vi "ABR-Init Hardware.vi"(0 "Params":T1={"Stimulus"={"Destination"="", "Waveform"=enum."TONE PIP", "Frequency (kHz)"=16.0, "Rep rate (/sec)"=30.0, "Alternate Polarity"=FALSE, "Sampling rate (Hz)"=0.0, "Duration (ms)"=30.0, "Ramp (ms)"=5.0, "Click width (us)"=0.0, "ITI"=enum."Rate"}, "Sequence"={"Start (dB)"=20, "Stop (dB)"=80, "Step (dB)"=5}, "Response"={"CAP or ABR"=enum."ABR", "Gain"=10000, "Averages"=512, "Window (ms)"=8.5, "Thr Fast Steps"=8.5, "Fs (Hz)"=25000.0, "Save raw"=FALSE}, "Normalize"=FALSE, "Reject"=0.0} {"Sequence"."Start (dB)" step=5; "Response"."Thr Fast Steps" format="%.2f"; "Response"."Window (ms)" format="%.2f"; "Stimulus"."Frequency (kHz)" format="%.2f"}, 11 "error in (no error)":errorcluster) -> (4 "Runtime":T5, 6 "AO npts":i32, 8 "Coerced rep rate":dbl, 15 "error out":errorcluster)   [LabVIEW 2020]
uses:
  Typedefs/ABR-Runtime Data.ctl
  epl-vi-lib/Signal Synthesis VIs/4th Generation/Classes/SignalManager/SignalManager.lvclass
  Typedefs/ABR-Parameters.ctl
  Typedefs/ABR-Stimulus.ctl
  Typedefs/ABR-Sequence.ctl
  Typedefs/ABR-Response.ctl
  5664aaa6-f0d2-4dbe-9bd7-bb78e569ca1b.vi
  6bfe4fab-d2cc-4fad-8abc-22872ba60b63.vi
  0f633bf1-3711-4c41-a985-7e54c01dc944.vi
  5e16f318-188a-4eb5-81ba-3342a0d43969.vi
  <vilib>/Utility/config.llb/Open Config Data.vi
  <vilib>/Utility/config.llb/Get Key Names.vi
  <vilib>/Utility/config.llb/Read Key.vi
  <vilib>/Utility/config.llb/Read Key (String).vi
  epl-vi-lib/Utility VIs/Array Manipulation VIs/String Array to Comma Separated String.vi
  <vilib>/Utility/error.llb/Error Cluster From Error Code.vi
  <vilib>/Utility/config.llb/Close Config Data.vi
  epl-vi-lib/PXI DAQ VIs/AODO/AODO-Engine.vi
  epl-vi-lib/PXI DAQ VIs/AIDI/AIDI-Engine.vi
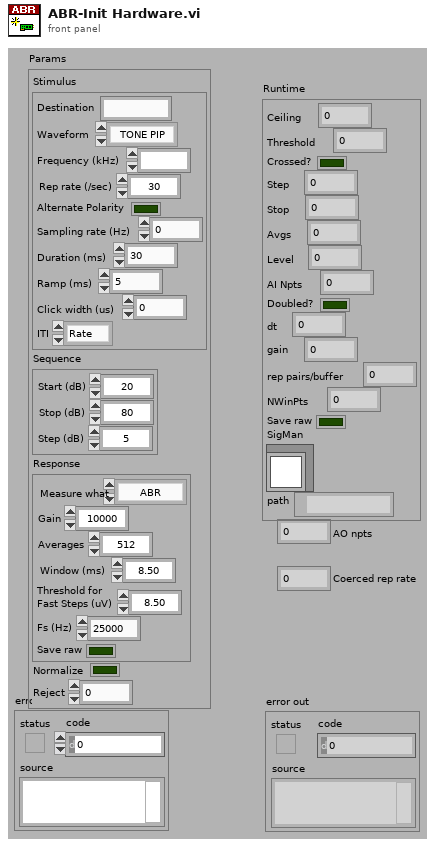
[diagram p1: front panel]
types:
  T1 = typedef "ABR-Parameters.ctl" = cluster{"Stimulus":T2, "Sequence":T3, "Response":T4, "Normalize":bool, "Reject":dbl}
  T2 = typedef "ABR-Stimulus.ctl" = cluster{"Destination":string, "Waveform":enum16{"TONE PIP", "CLICK"}, "Frequency (kHz)":ext, "Rep rate (/sec)":dbl, "Alternate Polarity":bool, "Sampling rate (Hz)":dbl, "Duration (ms)":dbl, "Ramp (ms)":dbl, "Click width (us)":dbl, "ITI":enum16{"Rate", "Interval"}}
  T3 = typedef "ABR-Sequence.ctl" = cluster{"Start (dB)":i32, "Stop (dB)":i32, "Step (dB)":i32}
  T4 = typedef "ABR-Response.ctl" = cluster{"CAP or ABR":enum16{"CAP", "ABR"}, "Gain":i32, "Averages":i32, "Window (ms)":sgl, "Thr Fast Steps":sgl, "Fs (Hz)":dbl, "Save raw":bool}
  T5 = typedef "ABR-Runtime Data.ctl" = cluster{"Ceiling":dbl, "Threshold":dbl, "Crossed?":bool, "Step":dbl, "Stop":i32, "Avgs":i32, "Level":dbl, "AI Npts":i32, "Doubled?":bool, "dt":dbl, "gain":dbl, "rep pairs/buffer":i32, "NWinPts":i32, "Save raw":bool, "SigMan":refnum<class "SignalManager.lvclass">, "path":path}
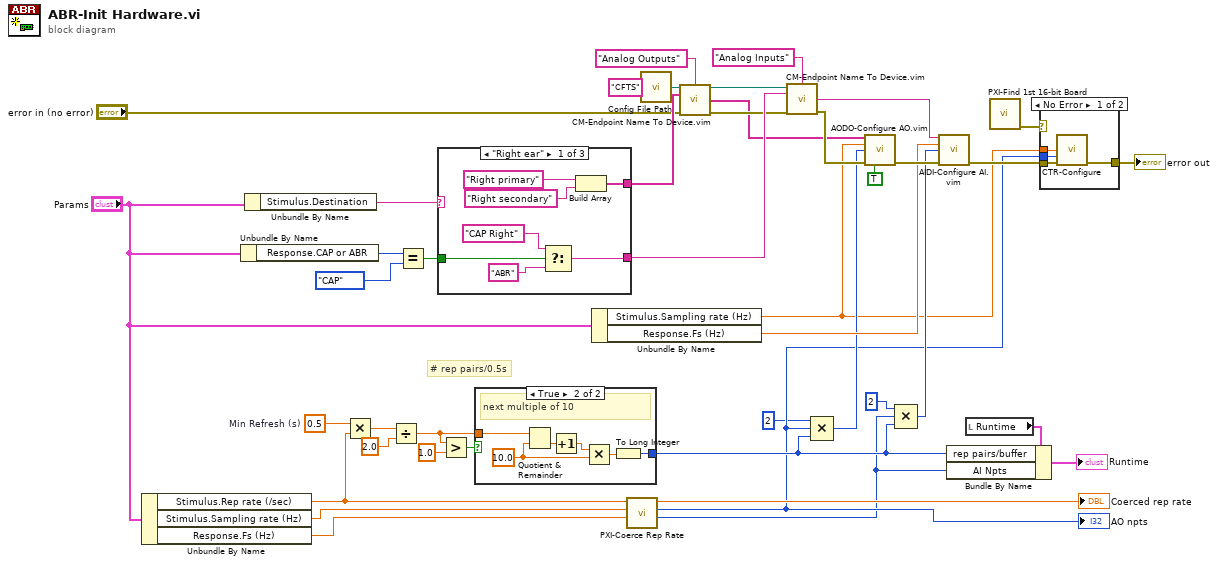
[diagram p0: block diagram]
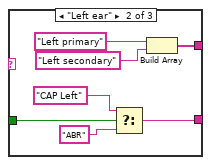
[diagram p3: hidden frame]
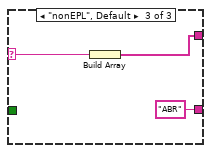
[diagram p4: hidden frame]
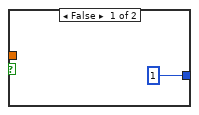
[diagram p5: hidden frame]
diagram:
  w35 = 0.5  # Min Refresh (s)
  # "# rep pairs/0.5s"
  n1 = Unbundle By Name("Params") -> ("Stimulus.Rep rate (/sec)"=w34:dbl, "Stimulus.Sampling rate (Hz)"=w14:dbl, "Response.Fs (Hz)"=w13:dbl)
  n2 = Unbundle By Name("Params") -> ("Response.CAP or ABR"=w31:enum16{"CAP", "ABR"})
  n3 = Unbundle By Name("Params") -> ("Stimulus.Destination"=w33:string)
  n4 = Multiply(x=w35, y=w34) -> (x*y=w36:dbl)
  n5 = Divide(x=w36, y=2.0) -> (x/y=w39:dbl)
  n6 = Equal?(x=w31, y=enum16{"CAP", "ABR"}."CAP") -> (x = y?=w29:bool)
  n7 = case shown="\"Right ear\"" w33 {
    selector: w33 -> [_ _ w60]
    tunnel: [w48 w55 w59] -> w23
    tunnel: w29 -> [w47 w54 _]
    tunnel: [w44 w51 "ABR"] -> w24
    frame "Right ear" {
      n8 = Select(t="CAP Right", s=w47, f="ABR") -> (s? t:f=w44:string)
      n9 = Build Array("Right primary", "Right secondary") -> (w48:string[])
    }
    frame "Left ear" {
      n10 = Select(t="CAP Left", s=w54, f="ABR") -> (s? t:f=w51:string)
      n11 = Build Array("Left primary", "Left secondary") -> (w55:string[])
    }
    frame "nonEPL", Default {
      n12 = Build Array(w60) -> (w59:string[])
    }
  }
  n13 = Greater?(x=w39, y=1.0) -> (0:w38:bool)
  n14 = case shown="True" w38 {
    tunnel: w39 -> [_ w67]
    tunnel: [1 w63] -> w11
    frame False {
    }
    frame True {
      w66 = 10.0 ("y")
      # "next multiple of 10"
      n15 = Quotient & Remainder(x=w67, y=w66) -> (floor(x/y)=w64:dbl)  [unwired: 1 out]
      n16 = Increment(x=w64) -> (x+1=w62:dbl)
      n17 = Multiply(x=w62, y=w66) -> (x*y=w65:dbl)
      n18 = To Long Integer(number=w65) -> (32bit integer=w63:i32)
    }
  }
  n19 = Unbundle By Name("Params") -> ("Stimulus.Sampling rate (Hz)"=w7:dbl, "Response.Fs (Hz)"=w15:dbl)
  n20 = call "PXI-Coerce Rep Rate.vi"("AI sampling rate (Hz)"=w13, "AO sampling rate (Hz)"=w14, "Rep rate (Hz)"=w34) -> ("AI npts"=w2:i32, "AO npts"=w6:i32, "Coerced rep rate (Hz)"=→"Coerced rep rate":dbl)  [unwired: 5 in, 1 out]
  "AO npts" <- w6
  n21 = call "Config File Path.vi"("AppName"="CFTS") -> ("Default config file name"=w28:path)
  n22 = call "CM-Endpoint Name To Device.vim"("Path"=w28, "IO Type"="Analog Outputs", "Names in"=w23, "error in (no error)"="error in (no error)") -> ("Path thru"=w25:path, "Devices"=w19:string[], "error out"=w21:errorcluster)  [unwired: 8 in, 1 out]
  n23 = call "CM-Endpoint Name To Device.vim"("Path"=w25, "IO Type"="Analog Inputs", "Names in"=w24, "error in (no error)"=w21) -> ("Devices"=w17:string, "error out"=w20:errorcluster)  [unwired: 8 in, 2 out]
  n24 = Compound Arithmetic op=MULTIPLY(2 ("value"), w6, w11) -> (w12:i32)
  n25 = call "AODO-Configure AO.vim"("AO.Channels"=w19, "AO.Fs (Hz)"=w7, "AO.Npts"=w12, "error in (no error)"=w20, "Allow regen? (F)"=TRUE ("Allow regen?")) -> ("error out"=w18:errorcluster)  [unwired: 10 in]
  n26 = Compound Arithmetic op=MULTIPLY(2 ("value"), w2, w11) -> (w10:i32)
  n27 = call "AIDI-Configure AI.vim"("AI.Channels"=w17, "AI.Fs (Hz)"=w15, "AI.Npts"=w10, "error in (no error)"=w18) -> ("error out"=w8:errorcluster)  [unwired: 11 in]
  n28 = local read "Runtime"() -> (w42:T5)
  n29 = Bundle By Name(cluster=w42, "rep pairs/buffer"=w11, "AI Npts"=w2) -> (→"Runtime":T5)
  n30 = call "PXI-Find 1st 16-bit Board.vi"() -> ("error out"=w1:errorcluster)  [unwired: 9 in, 2 out]
  n31 = case shown="No Error" w1 {
    tunnel: w8 -> [w71 w72]
    tunnel: w7 -> [w70 _]
    tunnel: w6 -> [w69 _]
    tunnel: [w68 w72] -> w5
    frame No Error {
      n32 = call "CTR-Configure.vi"("Sampling rate (Hz)"=w70, "Npts"=w69, "error in (no error)"=w71) -> ("error out"=w68:errorcluster)  [unwired: 12 in]
    }
    frame Error {
    }
  }
  "error out" <- w5
